vi "Get Localized Phrase Array.vi"(8 "error in":errorcluster, 9 "Target Language (current lang)":string, 10 "Keys":string[](array[string])) -> (0 "error out":errorcluster, 2 "Translated Phrases":string[](array[string]))   [LabVIEW 2019]
doc: "Gets the localized phrase by key from the current dictionary.\n\nKey: Unique identifier defined in the dictionary\nTarget Language (current lang): Optional input. Set this to translate a phase to a language other than the current language."
uses:
  SubVIs/Localization FGV Action -- Enum.ctl
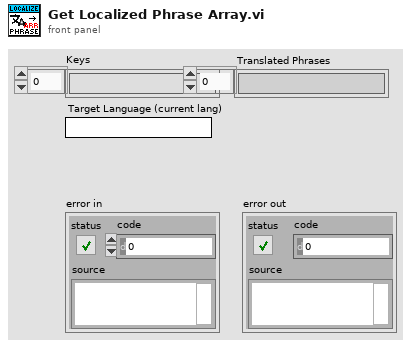
[diagram p1: front panel]
types:
  T1 = typedef "Localization FGV Action -- Enum.ctl" = enum16{"Read Dictionary", "Translate VIs", "Register VI", "Get Languages", "Translate Phrase", "Get Key For Phrase", "Get Phrase For Phrase", "Translate VI", "Unregister"}
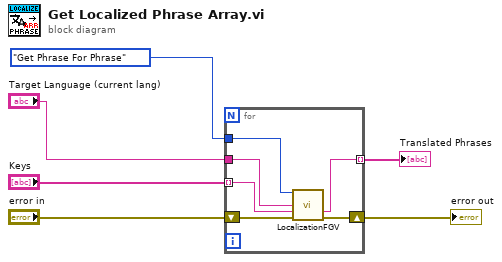
[diagram p0: block diagram]
diagram:
  n1 = for {
    tunnel: Localization_FGV_Action_--_Enum."Get Phrase For Phrase" ("Action") -> [w12]
    tunnel: "Keys" -> [w11] mode=indexing
    shift-right: [w8] -> w2
    shift-left: "error in" -> [w10]
    tunnel: "Target Language (current lang)" -> [w9]
    tunnel: [w7] -> w1 mode=indexing
    n2 = call "LocalizationFGV.vi"("Action"=w12, "Target Language"=w9, "Input"=w11, "error in"=w10) -> ("Result"=w7:string, "error out"=w8:errorcluster)  [unwired: 6 in, 4 out]
  }
  "error out" <- w2
  "Translated Phrases" <- w1
